vi "6.Photocell + LM35.vi"() -> ()   [LabVIEW 2014]
uses:
  <vilib>/LabVIEW Interface for Arduino/Type Defs/Connection Type.ctl
  <vilib>/LabVIEW Interface for Arduino/Type Defs/Board Type.ctl
  <vilib>/LabVIEW Interface for Arduino/LabVIEW Interface for Arduino.lvlib
panel:
  in  "Stop":bool
  out "Tab Control":enum32{"Temp Sensor", "Light Sensor"}(tab)
  out "Voltage":dbl(knob) scale=0.0..5.0
  in  "VISA resource":refnum<visa-resource-name>
  in  "LM35 Pin (0)":u8
  out "Temperature(deg)":dbl(slide) scale=0.0..100.0
  out "Fahrenheit(*F)":dbl
  out "Time String":string
  out "Light Intensity":dbl(knob) scale=0.0..100.0
  in  "Photo Cell Pin (0)":u8
  out "Waveform Chart":dbl(graph)
  in  "Time Stamp":timestamp
  out "date string":string
  # "Stop"
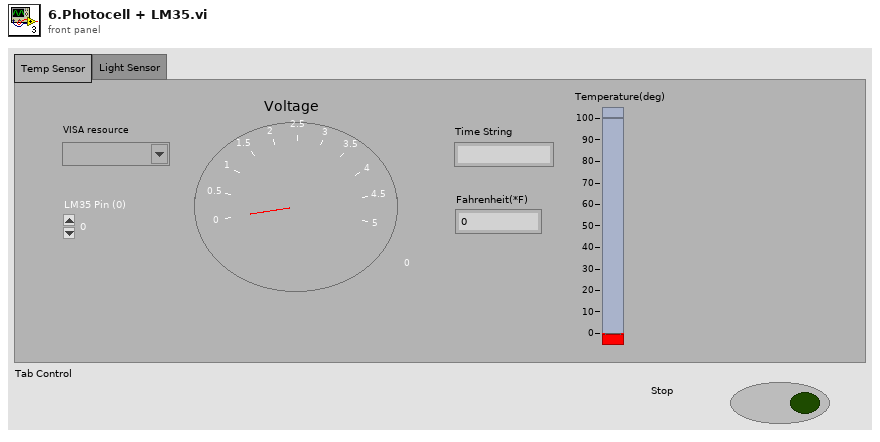
[diagram p1: front panel]
types:
  T1 = typedef "LabVIEW Interface for Arduino.lvlib/Board Type.ctl" = enum16{"Uno", "Dimuelanove w/Atmega 328", "Mega 2560"}
  T2 = typedef "LabVIEW Interface for Arduino.lvlib/Connection Type.ctl" = enum8{"USB / Serial", "XBEE", "BlueSmirf (Bluetooth)"}
  T3 = typedef "LabVIEW Interface for Arduino.lvlib/Arduino Resource.ctl" = cluster{"VISA resource":refnum<visa-resource-name>, "Board Type":T1, "Connection Type":enum8{"USB / Serial"}, "Bytes Per Packet (15)":u8}
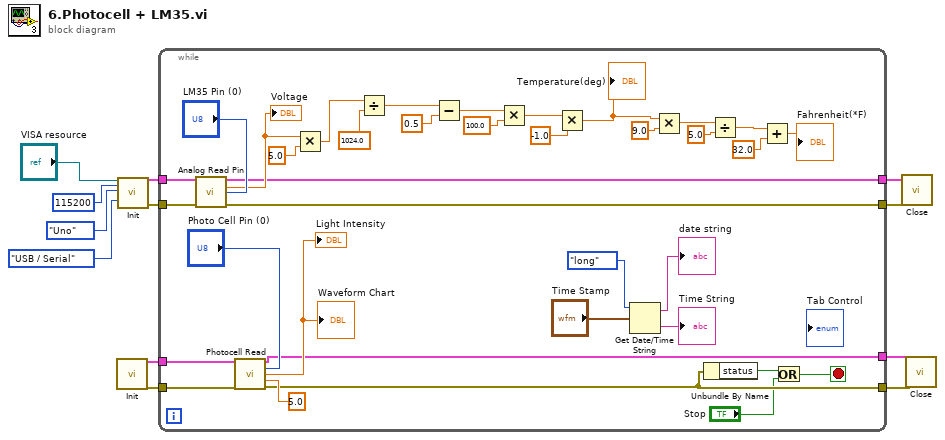
[diagram p0: block diagram]
diagram:
  n1 = call <vilib>:"Init.vi"() -> ("Arduino Resource"=w8:T3, "error out"=w7:errorcluster)  [unwired: 18 in]
  n2 = call <vilib>:"Init.vi"("VISA resource"="VISA resource", "Baud Rate (115200)"=u32 115200, "Board Type (Uno)"=Board_Type."Uno", "Connection Type (USB/Serial)"=Connection_Type."USB / Serial") -> ("Arduino Resource"=w1:T3, "error out"=w2:errorcluster)  [unwired: 14 in]
  n3 = while {
    tunnel: w8 -> [w23]
    tunnel: w7 -> [w26]
    tunnel: [w25] -> w4
    tunnel: [w22] -> w3
    tunnel: [w17] -> w6
    tunnel: [w16] -> w5
    tunnel: w2 -> [w15]
    tunnel: w1 -> [w14]
    stop <- w28 stop-if-true
    n4 = call <vilib>:"Analog Read Pin.vi"("Arduino Resource"=w14, "Analog Input Pin (0)"="LM35 Pin (0)", "error in"=w15) -> ("Arduino Resource"=w17:T3, "Voltage"=w44:dbl, "error out"=w16:errorcluster)  [unwired: 10 in]
    "Voltage" <- w44
    n5 = call <vilib>:"Photocell Read.vi"("Arduino Resource"=w23, "Photo Cell Pin (0)"="Photo Cell Pin (0)", "Vcc (5)"=5.0, "error in"=w26) -> ("Arduino Resource"=w22:T3, "Light Intensity (0 - 100)"=→"Waveform Chart" →"Light Intensity":dbl, "error out"=w25:errorcluster)  [unwired: 9 in]
    n6 = Multiply(x=w44, y=5.0) -> (x*y=w43:dbl)
    n7 = Divide(x=w43, y=1024.0) -> (x/y=w24:dbl)
    n8 = Subtract(x=w24, y=0.5) -> (x-y=w41:dbl)
    n9 = Multiply(x=w41, y=100.0) -> (x*y=w19:dbl)
    n10 = Multiply(x=w19, y=-1.0) -> (x*y=w21:dbl)
    "Temperature(deg)" <- w21
    n11 = Get Date/Time String(date format (0)=enum16{"short", "long", "abbreviated"}."long", seconds (now)="Time Stamp") -> (date string=→"date string":string, time string=→"Time String":string)  [unwired: 1 in]
    n12 = Multiply(x=w21, y=9.0) -> (x*y=w38:dbl)
    n13 = Unbundle By Name(w25) -> ("status"=w29:bool)
    n14 = Divide(x=w38, y=5.0) -> (x/y=w36:dbl)
    n15 = Add(x=w36, y=32.0) -> (x+y=→"Fahrenheit(*F)":dbl)
    n16 = Or(x=w29, y="Stop") -> (x .or. y?=w28:bool)
  }
  n17 = call <vilib>:"Close.vi"("Arduino Resource"=w6, "error in"=w5) -> ()  [unwired: 13 in, 1 out]
  n18 = call <vilib>:"Close.vi"("Arduino Resource"=w3, "error in"=w4) -> ()  [unwired: 13 in, 1 out]
